vi "ConnectFieldTestServer.vi"(0 "FileName(.txt)":string="Test", 1 "working directory":path=path "C:/RageATE-Pickerel/Automated Tests/Tetra_RFSM/support_files/FieldTestServer", 5 "error in (no error)":errorcluster, 6 "UseCmdFile(T)":bool, 7 "Skip(T)":bool, 11 "CmdWindowHide(T)":bool, 13 "OpenNewFt(T)":bool=TRUE) -> (10 "PID":string="3196", 12 "cmd_path_out":path=path "C:/RageATE-Pickerel/Automated Tests/Tetra_RFSM/support_files/FieldTestServer/cmd /c FieldTest.exe testConfig_RfsmOnly.scn > Test.txt", 14 "success?(t)":bool=TRUE, 16 "connectToFt":string, 17 "cctFt error":string, 18 "cctFt output":string, 19 "error out":errorcluster)   [LabVIEW 2018]
panel:
  out "FtSvcOpen?(t)":bool
  out "KillFT(t)":bool caption="OK"
  out "FieldTestOpen?(t)":bool
  out "standard output":string="INFO: No tasks are running which match the specified criteria.Image Name                     PID Services                                    \r\n========================= ======== ============================================\r\nSystem Idle Process              0 N/A                                         \r\nSystem                           4 N/A                                         \r\nRegistry                       124 N/A                                         \r\nsmss.exe                       452 N/A                                         \r\ncsrss.exe                      592 N/A                                         \r\nwininit.exe                    792 N/A                                         \r\ncsrss.exe                      800 N/A                                         \r\nservices.exe                   880 N/A                                         \r\nlsass.exe                      888 KeyIso, SamSs, VaultSvc                     \r\nsvchost.exe                     84 BrokerInfrastructure, DcomLaunch, PlugPlay, \r\n                                   Power, SystemEventsBroker                   \r\nfontdrvhost.exe                536 N/A                                         \r\nwinlogon.exe                   664 N/A                                         \r\nfontdrvhost.exe                732 N/A                                         \r\nsvchost.exe                    964 RpcEptMapper, RpcSs                         \r\nsvchost.exe                    708 LSM                                         \r\ndwm.exe                       1080 N/A                                         \r\nsvchost.exe                   1276 NcbService                                  \r\nsvchost.exe                   1316 lmhosts                                     \r\nsvchost.exe                   1324 TimeBrokerSvc                               \r\nsvchost.exe                   1388 EventLog                                    \r\nsvchost.exe                   1396 hidserv                                     \r\nsvchost.exe                   1544 DevQueryBroker                              \r\nsvchost.exe                   1552 nsi                                         \r\nsvchost.exe                   1608 Dhcp                                        \r\nNVDisplay.Container.exe       1736 NVDisplay.ContainerLocalSystem              \r\nsvchost.exe                   1752 NlaSvc                                      \r\nsvchost.exe                   1812 Schedule                                    \r\nsvchost.exe                   1900 ProfSvc                                     \r\nsvchost.exe                   1908 SysMain                                     \r\nsvchost.exe                   1916 Themes                                      \r\nsvchost.exe                   1924 netprofm                                    \r\nsvchost.exe                   1940 EventSystem                                 \r\nsvchost.exe                   2052 SENS                                        \r\nsvchost.exe                   2076 AudioEndpointBuilder                        \r\nsvchost.exe                   2084 FontCache                                   \r\nMemory Compression            2144 N/A                                         \r\nsvchost.exe                   2456 WinHttpAutoProxySvc                         \r\nsvchost.exe                   2472 UserManager                                 \r\nsvchost.exe                   2532 Dnscache                                    \r\nsvchost.exe                   2612 Audiosrv                                    \r\nsvchost.exe                   2664 Wcmsvc                                      \r\nsvchost.exe                   2672 DusmSvc                                     \r\nsvchost.exe                   2736 ShellHWDetection                            \r\nspoolsv.exe                   2912 Spooler                                     \r\nsvchost.exe                   2956 BFE, mpssvc                                 \r\nsvchost.exe                   2996 StateRepository                             \r\nsvchost.exe                   3032 LanmanWorkstation                           \r\nsvchost.exe                   3260 CoreMessagingRegistrar                      \r\nsvchost.exe                   3268 CryptSvc                                    \r\nsvchost.exe                   3276 TermService                                 \r\nsvchost.exe                   3284 Winmgmt                                     \r\nsvchost.exe                   3292 DiagTrack                                   \r\nsvchost.exe                   3300 DPS                                         \r\nsvchost.exe                   3308 WpnService                                  \r\nIOLibrariesService.exe        3316 IOLibrariesService                          \r\nsvchost.exe                   3332 TrkWks                                      \r\nsvchost.exe                   3340 stisvc                                      \r\nnipalsm.exe                   3352 ni488enumsvc                                \r\nnimxs.exe                     3360 mxssvr                                      \r\nsvchost.exe                   3372 SstpSvc                                     \r\nKeysightCommunicationsFab     3380 KeysightCommunicationsFabric                \r\nLegacyDiscoveryService.ex     3392 AgilentInstrumentDiscoveryService           \r\nsvchost.exe                   3408 DeviceAssociationService                    \r\nLxiMdnsResponder.exe          3416 AgtMdnsResponder                            \r\nKeysightInstrumentIoServi     3460 KeysightInstrumentIoService                 \r\nnisvcloc.exe                  3484 NiSvcLoc                                    \r\ntvnserver.exe                 3496 tvnserver                                   \r\nnipxicms.exe                  3508 nipxicmsvc                                  \r\nnisds.exe                     3536 nisds                                       \r\narmsvc.exe                    3548 AdobeARMservice                             \r\nMsMpEng.exe                   3556 WinDefend                                   \r\nvss-service-x64.exe           3568 Synology Drive VSS Service x64              \r\nniauth_daemon.exe             3588 niauth                                      \r\nOfficeClickToRun.exe          3772 ClickToRunSvc                               \r\nsvchost.exe                   3808 WdiServiceHost                              \r\ndasHost.exe                   3940 N/A                                         \r\nsvchost.exe                   3984 iphlpsvc                                    \r\nHppSupportService.exe         4036 HppSupportService                           \r\nAgilentLicenseService.exe     4044 Agilent License Service                     \r\nsvchost.exe                   4076 LanmanServer                                \r\nsvchost.exe                   3976 RasMan                                      \r\nkiis-service.exe              4372 N/A                                         \r\nconhost.exe                   4388 N/A                                         \r\nsvchost.exe                   4748 SSDPSRV                                     \r\nlkads.exe                     4800 lkClassAds                                  \r\nniroco.exe                    4808 niroco                                      \r\nlktsrv.exe                    4964 lkTimeSync                                  \r\nnipxism.exe                   4972 nipxirmu                                    \r\nnidmsrv.exe                   4992 NIDomainService                             \r\nnimdnsResponder.exe           5008 nimDNSResponder                             \r\nnidevldu.exe                  5124 nidevldu                                    \r\ntagsrv.exe                    5184 NITaggerService                             \r\nniLxiDiscovery.exe            5252 niLXIDiscovery                              \r\nniDiscSvc.exe                 5276 NINetworkDiscovery                          \r\nsvchost.exe                   5452 PolicyAgent                                 \r\ndasHost.exe                   6020 N/A                                         \r\nLegacyIOLibrariesService.     6084 AgilentIOLibrariesService                   \r\nConnectionExpert.Server.H     6092 KeysightInstrumentDiscoveryService          \r\nSystemWebServer.exe           6108 NISystemWebServer                           \r\nApplicationWebServer.exe      6564 NIApplicationWebServer                      \r\nNIWebServiceContainer.exe     6572 N/A                                         \r\nNIWebServiceContainer.exe     6648 N/A                                         \r\nNIWebServiceContainer.exe     6708 N/A                                         \r\nNIWebServiceContainer.exe     6776 N/A                                         \r\nsvchost.exe                   7132 DispBrokerDesktopSvc                        \r\nsvchost.exe                   6716 NcdAutoSetup                                \r\nsvchost.exe                   6916 FDResPub                                    \r\nNIWebServiceContainer.exe     6060 N/A                                         \r\nIolsNkoServer.exe             2908 N/A                                         \r\nSearchIndexer.exe             6980 WSearch                                     \r\niproc488.exe                  7688 N/A                                         \r\niproc82357.exe                7764 N/A                                         \r\niproc389.exe                  7800 N/A                                         \r\nsecure-config-service.exe     7844 N/A                                         \r\nconhost.exe                   7852 N/A                                         \r\nAggregatorHost.exe            7504 N/A                                         \r\nIolsPXIResourceManager.ex     8104 IolsPXIResourceManager                      \r\nsecurity-comm-hpp-microse     7252 N/A                                         \r\nconhost.exe                   7296 N/A                                         \r\ndllhost.exe                   8820 N/A                                         \r\nNisSrv.exe                    9092 WdNisSvc                                    \r\nsvchost.exe                   8212 WdiSystemHost                               \r\nsvchost.exe                   7508 PcaSvc                                      \r\nNVDisplay.Container.exe       9456 N/A                                         \r\nsvchost.exe                   2932 DoSvc                                       \r\nsvchost.exe                   7572 RmSvc                                       \r\nsvchost.exe                   1420 StorSvc                                     \r\nsvchost.exe                   9584 NgcSvc                                      \r\nsvchost.exe                   9784 NgcCtnrSvc                                  \r\nsvchost.exe                   9676 CertPropSvc                                 \r\nsvchost.exe                   9640 SCardSvr                                    \r\nsvchost.exe                   2564 CDPSvc                                      \r\nSgrmBroker.exe                1568 SgrmBroker                                  \r\nuhssvc.exe                    2040 uhssvc                                      \r\nsvchost.exe                   2604 TokenBroker                                 \r\nsvchost.exe                   2936 UsoSvc                                      \r\nsvchost.exe                   3600 W32Time                                     \r\nsvchost.exe                   4356 wscsvc                                      \r\nsvchost.exe                   1288 InstallService                              \r\nsihost.exe                    8492 N/A                                         \r\nsvchost.exe                   9356 CDPUserSvc_5dc012                           \r\nsvchost.exe                    896 WpnUserService_5dc012                       \r\ntaskhostw.exe                 4328 N/A                                         \r\nsvchost.exe                   2420 TabletInputService                          \r\nctfmon.exe                    2864 N/A                                         \r\nexplorer.exe                  2108 N/A                                         \r\nsvchost.exe                   7040 camsvc                                      \r\nsvchost.exe                   9196 cbdhsvc_5dc012                              \r\nStartMenuExperienceHost.e      704 N/A                                         \r\nRuntimeBroker.exe             2356 N/A                                         \r\nSearchApp.exe                10092 N/A                                         \r\nRuntimeBroker.exe             8364 N/A                                         \r\nsvchost.exe                   8024 LicenseManager                              \r\nRuntimeBroker.exe            11248 N/A                                         \r\nsvchost.exe                  10560 OneSyncSvc_5dc012,                          \r\n                                   PimIndexMaintenanceSvc_5dc012,              \r\n                                   UnistoreSvc_5dc012, UserDataSvc_5dc012      \r\nPhoneExperienceHost.exe       9244 N/A                                         \r\ndllhost.exe                  11364 N/A                                         \r\nRuntimeBroker.exe            11520 N/A                                         \r\nTextInputHost.exe            11604 N/A                                         \r\nSecurityHealthSystray.exe    11752 N/A                                         \r\nSecurityHealthService.exe    11784 SecurityHealthService                       \r\ntvnserver.exe                11908 N/A                                         \r\nsvchost.exe                  12676 Appinfo                                     \r\nms-teams.exe                  9444 N/A                                         \r\nRuntimeBroker.exe             6580 N/A                                         \r\niprocsvr.exe                  7308 N/A                                         \r\niproc8491.exe                 6028 N/A                                         \r\nAgilentLicenseNotifier.ex    12968 N/A                                         \r\nDeviceMonitor.exe            13488 N/A                                         \r\nmsedgewebview2.exe           13624 N/A                                         \r\ndllhost.exe                  13660 N/A                                         \r\nmsedgewebview2.exe           13680 N/A                                         \r\nmsedgewebview2.exe           13996 N/A                                         \r\nmsedgewebview2.exe           14016 N/A                                         \r\nmsedgewebview2.exe           14040 N/A                                         \r\nmsedgewebview2.exe           14156 N/A                                         \r\nnierserver.exe               13372 N/A                                         \r\ncloud-drive-ui.exe           15264 N/A                                         \r\ncloud-drive-connect.exe       8788 N/A                                         \r\nconhost.exe                  14372 N/A                                         \r\ncloud-drive-daemon.exe       15008 N/A                                         \r\nconhost.exe                  15052 N/A                                         \r\nmsedgewebview2.exe           14456 N/A                                         \r\nsvchost.exe                  14524 lfsvc                                       \r\nApplicationFrameHost.exe     12392 N/A                                         \r\nCalculatorApp.exe            12440 N/A                                         \r\nRuntimeBroker.exe             3492 N/A                                         \r\nSystemSettings.exe            3580 N/A                                         \r\nUserOOBEBroker.exe           12412 N/A                                         \r\nMicrosoft.Media.Player.ex     6192 N/A                                         \r\nRuntimeBroker.exe             1724 N/A                                         \r\nOUTLOOK.EXE                   3908 N/A                                         \r\nai.exe                       10320 N/A                                         \r\nmsedgewebview2.exe            9184 N/A                                         \r\nmsedgewebview2.exe            2492 N/A                                         \r\nmsedgewebview2.exe            3016 N/A                                         \r\nmsedgewebview2.exe            1368 N/A                                         \r\nmsedgewebview2.exe           10564 N/A                                         \r\nmsedgewebview2.exe            7120 N/A                                         \r\nmsedgewebview2.exe           12888 N/A                                         \r\nfirefox.exe                  13096 N/A                                         \r\nfirefox.exe                  12984 N/A                                         \r\nfirefox.exe                  13228 N/A                                         \r\nfirefox.exe                   7624 N/A                                         \r\nfirefox.exe                   6244 N/A                                         \r\nfirefox.exe                  15312 N/A                                         \r\nfirefox.exe                    820 N/A                                         \r\nTGitCache.exe                 5360 N/A                                         \r\nsvchost.exe                  14784 wcncsvc                                     \r\nShellExperienceHost.exe      12404 N/A                                         \r\nRuntimeBroker.exe             6468 N/A                                         \r\nVideo.UI.exe                 13360 N/A                                         \r\nRuntimeBroker.exe            13412 N/A                                         \r\nsvchost.exe                   5304 BthAvctpSvc                                 \r\nsvchost.exe                   1264 WebClient                                   \r\nWinRAR.exe                   15756 N/A                                         \r\nmsedge.exe                    9240 N/A                                         \r\nmsedge.exe                   16444 N/A                                         \r\nmsedge.exe                   15112 N/A                                         \r\nmsedge.exe                   15656 N/A                                         \r\nmsedge.exe                    9208 N/A                                         \r\nmsedge.exe                    9068 N/A                                         \r\nmsedge.exe                   16896 N/A                                         \r\nmsedge.exe                   10192 N/A                                         \r\nmsedge.exe                   10844 N/A                                         \r\nmsedge.exe                    1432 N/A                                         \r\nmsedge.exe                   12940 N/A                                         \r\nmsedge.exe                    1652 N/A                                         \r\nmsedge.exe                    9800 N/A                                         \r\nmsedge.exe                   13316 N/A                                         \r\nmsedge.exe                   15800 N/A                                         \r\nmsedge.exe                   11328 N/A                                         \r\nmsedge.exe                    1808 N/A                                         \r\nfirefox.exe                  17812 N/A                                         \r\nfirefox.exe                  17620 N/A                                         \r\nfirefox.exe                  14588 N/A                                         \r\nmsedge.exe                   11468 N/A                                         \r\nai.exe                       15952 N/A                                         \r\nmsedge.exe                    5872 N/A                                         \r\nmsedge.exe                   10824 N/A                                         \r\nSnippingTool.exe              4636 N/A                                         \r\ntvnviewer.exe                18856 N/A                                         \r\nfirefox.exe                  14060 N/A                                         \r\nfirefox.exe                   2116 N/A                                         \r\nfirefox.exe                  10568 N/A                                         \r\nfirefox.exe                  15436 N/A                                         \r\nfirefox.exe                  10688 N/A                                         \r\nfirefox.exe                  15292 N/A                                         \r\nfirefox.exe                  19384 N/A                                         \r\nfirefox.exe                   1412 N/A                                         \r\nsvchost.exe                  15940 DsSvc                                       \r\nfirefox.exe                   3848 N/A                                         \r\nfirefox.exe                  12172 N/A                                         \r\nfirefox.exe                  10924 N/A                                         \r\naudiodg.exe                   9120 N/A                                         \r\nOneDrive.exe                  9532 N/A                                         \r\nMicrosoft.SharePoint.exe     15608 N/A                                         \r\nFileCoAuth.exe               13268 N/A                                         \r\nLabVIEW.exe                  17668 N/A                                         \r\nnimxsoffline.exe             10864 N/A                                         \r\nfirefox.exe                  18416 N/A                                         \r\nfirefox.exe                  12188 N/A                                         \r\nWmiPrvSE.exe                 17864 N/A                                         \r\nsvchost.exe                  17244 gpsvc                                       \r\nsmartscreen.exe              17352 N/A                                         \r\nSearchProtocolHost.exe        3472 N/A                                         \r\nSearchFilterHost.exe         12868 N/A                                         \r\ntasklist.exe                 19020 N/A                                         \r\nconhost.exe                  18652 N/AImage Name                     PID Services                                    \r\n========================= ======== ============================================\r\nSystem Idle Process              0 N/A                                         \r\nSystem                           4 N/A                                         \r\nRegistry                       124 N/A                                         \r\nsmss.exe                       452 N/A                                         \r\ncsrss.exe                      592 N/A                                         \r\nwininit.exe                    792 N/A                                         \r\ncsrss.exe                      800 N/A                                         \r\nservices.exe                   880 N/A                                         \r\nlsass.exe                      888 KeyIso, SamSs, VaultSvc                     \r\nsvchost.exe                     84 BrokerInfrastructure, DcomLaunch, PlugPlay, \r\n                                   Power, SystemEventsBroker                   \r\nfontdrvhost.exe                536 N/A                                         \r\nwinlogon.exe                   664 N/A                                         \r\nfontdrvhost.exe                732 N/A                                         \r\nsvchost.exe                    964 RpcEptMapper, RpcSs                         \r\nsvchost.exe                    708 LSM                                         \r\ndwm.exe                       1080 N/A                                         \r\nsvchost.exe                   1276 NcbService                                  \r\nsvchost.exe                   1316 lmhosts                                     \r\nsvchost.exe                   1324 TimeBrokerSvc                               \r\nsvchost.exe                   1388 EventLog                                    \r\nsvchost.exe                   1396 hidserv                                     \r\nsvchost.exe                   1544 DevQueryBroker                              \r\nsvchost.exe                   1552 nsi                                         \r\nsvchost.exe                   1608 Dhcp                                        \r\nNVDisplay.Container.exe       1736 NVDisplay.ContainerLocalSystem              \r\nsvchost.exe                   1752 NlaSvc                                      \r\nsvchost.exe                   1812 Schedule                                    \r\nsvchost.exe                   1900 ProfSvc                                     \r\nsvchost.exe                   1908 SysMain                                     \r\nsvchost.exe                   1916 Themes                                      \r\nsvchost.exe                   1924 netprofm                                    \r\nsvchost.exe                   1940 EventSystem                                 \r\nsvchost.exe                   2052 SENS                                        \r\nsvchost.exe                   2076 AudioEndpointBuilder                        \r\nsvchost.exe                   2084 FontCache                                   \r\nMemory Compression            2144 N/A                                         \r\nsvchost.exe                   2456 WinHttpAutoProxySvc                         \r\nsvchost.exe                   2472 UserManager                                 \r\nsvchost.exe                   2532 Dnscache                                    \r\nsvchost.exe                   2612 Audiosrv                                    \r\nsvchost.exe                   2664 Wcmsvc                                      \r\nsvchost.exe                   2672 DusmSvc                                     \r\nsvchost.exe                   2736 ShellHWDetection                            \r\nspoolsv.exe                   2912 Spooler                                     \r\nsvchost.exe                   2956 BFE, mpssvc                                 \r\nsvchost.exe                   2996 StateRepository                             \r\nsvchost.exe                   3032 LanmanWorkstation                           \r\nsvchost.exe                   3260 CoreMessagingRegistrar                      \r\nsvchost.exe                   3268 CryptSvc                                    \r\nsvchost.exe                   3276 TermService                                 \r\nsvchost.exe                   3284 Winmgmt                                     \r\nsvchost.exe                   3292 DiagTrack                                   \r\nsvchost.exe                   3300 DPS                                         \r\nsvchost.exe                   3308 WpnService                                  \r\nIOLibrariesService.exe        3316 IOLibrariesService                          \r\nsvchost.exe                   3332 TrkWks                                      \r\nsvchost.exe                   3340 stisvc                                      \r\nnipalsm.exe                   3352 ni488enumsvc                                \r\nnimxs.exe                     3360 mxssvr                                      \r\nsvchost.exe                   3372 SstpSvc                                     \r\nKeysightCommunicationsFab     3380 KeysightCommunicationsFabric                \r\nLegacyDiscoveryService.ex     3392 AgilentInstrumentDiscoveryService           \r\nsvchost.exe                   3408 DeviceAssociationService                    \r\nLxiMdnsResponder.exe          3416 AgtMdnsResponder                            \r\nKeysightInstrumentIoServi     3460 KeysightInstrumentIoService                 \r\nnisvcloc.exe                  3484 NiSvcLoc                                    \r\ntvnserver.exe                 3496 tvnserver                                   \r\nnipxicms.exe                  3508 nipxicmsvc                                  \r\nnisds.exe                     3536 nisds                                       \r\narmsvc.exe                    3548 AdobeARMservice                             \r\nMsMpEng.exe                   3556 WinDefend                                   \r\nvss-service-x64.exe           3568 Synology Drive VSS Service x64              \r\nniauth_daemon.exe             3588 niauth                                      \r\nOfficeClickToRun.exe          3772 ClickToRunSvc                               \r\nsvchost.exe                   3808 WdiServiceHost                              \r\ndasHost.exe                   3940 N/A                                         \r\nsvchost.exe                   3984 iphlpsvc                                    \r\nHppSupportService.exe         4036 HppSupportService                           \r\nAgilentLicenseService.exe     4044 Agilent License Service                     \r\nsvchost.exe                   4076 LanmanServer                                \r\nsvchost.exe                   3976 RasMan                                      \r\nkiis-service.exe              4372 N/A                                         \r\nconhost.exe                   4388 N/A                                         \r\nsvchost.exe                   4748 SSDPSRV                                     \r\nlkads.exe                     4800 lkClassAds                                  \r\nniroco.exe                    4808 niroco                                      \r\nlktsrv.exe                    4964 lkTimeSync                                  \r\nnipxism.exe                   4972 nipxirmu                                    \r\nnidmsrv.exe                   4992 NIDomainService                             \r\nnimdnsResponder.exe           5008 nimDNSResponder                             \r\nnidevldu.exe                  5124 nidevldu                                    \r\ntagsrv.exe                    5184 NITaggerService                             \r\nniLxiDiscovery.exe            5252 niLXIDiscovery                              \r\nniDiscSvc.exe                 5276 NINetworkDiscovery                          \r\nsvchost.exe                   5452 PolicyAgent                                 \r\ndasHost.exe                   6020 N/A                                         \r\nLegacyIOLibrariesService.     6084 AgilentIOLibrariesService                   \r\nConnectionExpert.Server.H     6092 KeysightInstrumentDiscoveryService          \r\nSystemWebServer.exe           6108 NISystemWebServer                           \r\nApplicationWebServer.exe      6564 NIApplicationWebServer                      \r\nNIWebServiceContainer.exe     6572 N/A                                         \r\nNIWebServiceContainer.exe     6648 N/A                                         \r\nNIWebServiceContainer.exe     6708 N/A                                         \r\nNIWebServiceContainer.exe     6776 N/A                                         \r\nsvchost.exe                   7132 DispBrokerDesktopSvc                        \r\nsvchost.exe                   6716 NcdAutoSetup                                \r\nsvchost.exe                   6916 FDResPub                                    \r\nNIWebServiceContainer.exe     6060 N/A                                         \r\nIolsNkoServer.exe             2908 N/A                                         \r\nSearchIndexer.exe             6980 WSearch                                     \r\niproc488.exe                  7688 N/A                                         \r\niproc82357.exe                7764 N/A                                         \r\niproc389.exe                  7800 N/A                                         \r\nsecure-config-service.exe     7844 N/A                                         \r\nconhost.exe                   7852 N/A                                         \r\nAggregatorHost.exe            7504 N/A                                         \r\nIolsPXIResourceManager.ex     8104 IolsPXIResourceManager                      \r\nsecurity-comm-hpp-microse     7252 N/A                                         \r\nconhost.exe                   7296 N/A                                         \r\ndllhost.exe                   8820 N/A                                         \r\nNisSrv.exe                    9092 WdNisSvc                                    \r\nsvchost.exe                   8212 WdiSystemHost                               \r\nsvchost.exe                   7508 PcaSvc                                      \r\nNVDisplay.Container.exe       9456 N/A                                         \r\nsvchost.exe                   2932 DoSvc                                       \r\nsvchost.exe                   7572 RmSvc                                       \r\nsvchost.exe                   1420 StorSvc                                     \r\nsvchost.exe                   9584 NgcSvc                                      \r\nsvchost.exe                   9784 NgcCtnrSvc                                  \r\nsvchost.exe                   9676 CertPropSvc                                 \r\nsvchost.exe                   9640 SCardSvr                                    \r\nsvchost.exe                   2564 CDPSvc                                      \r\nSgrmBroker.exe                1568 SgrmBroker                                  \r\nuhssvc.exe                    2040 uhssvc                                      \r\nsvchost.exe                   2604 TokenBroker                                 \r\nsvchost.exe                   2936 UsoSvc                                      \r\nsvchost.exe                   3600 W32Time                                     \r\nsvchost.exe                   4356 wscsvc                                      \r\nsvchost.exe                   1288 InstallService                              \r\nsihost.exe                    8492 N/A                                         \r\nsvchost.exe                   9356 CDPUserSvc_5dc012                           \r\nsvchost.exe                    896 WpnUserService_5dc012                       \r\ntaskhostw.exe                 4328 N/A                                         \r\nsvchost.exe                   2420 TabletInputService                          \r\nctfmon.exe                    2864 N/A                                         \r\nexplorer.exe                  2108 N/A                                         \r\nsvchost.exe                   7040 camsvc                                      \r\nsvchost.exe                   9196 cbdhsvc_5dc012                              \r\nStartMenuExperienceHost.e      704 N/A                                         \r\nRuntimeBroker.exe             2356 N/A                                         \r\nSearchApp.exe                10092 N/A                                         \r\nRuntimeBroker.exe             8364 N/A                                         \r\nsvchost.exe                   8024 LicenseManager                              \r\nRuntimeBroker.exe            11248 N/A                                         \r\nsvchost.exe                  10560 OneSyncSvc_5dc012,                          \r\n                                   PimIndexMaintenanceSvc_5dc012,              \r\n                                   UnistoreSvc_5dc012, UserDataSvc_5dc012      \r\nPhoneExperienceHost.exe       9244 N/A                                         \r\ndllhost.exe                  11364 N/A                                         \r\nRuntimeBroker.exe            11520 N/A                                         \r\nTextInputHost.exe            11604 N/A                                         \r\nSecurityHealthSystray.exe    11752 N/A                                         \r\nSecurityHealthService.exe    11784 SecurityHealthService                       \r\ntvnserver.exe                11908 N/A                                         \r\nsvchost.exe                  12676 Appinfo                                     \r\nms-teams.exe                  9444 N/A                                         \r\nRuntimeBroker.exe             6580 N/A                                         \r\niprocsvr.exe                  7308 N/A                                         \r\niproc8491.exe                 6028 N/A                                         \r\nAgilentLicenseNotifier.ex    12968 N/A                                         \r\nDeviceMonitor.exe            13488 N/A                                         \r\nmsedgewebview2.exe           13624 N/A                                         \r\ndllhost.exe                  13660 N/A                                         \r\nmsedgewebview2.exe           13680 N/A                                         \r\nmsedgewebview2.exe           13996 N/A                                         \r\nmsedgewebview2.exe           14016 N/A                                         \r\nmsedgewebview2.exe           14040 N/A                                         \r\nmsedgewebview2.exe           14156 N/A                                         \r\nnierserver.exe               13372 N/A                                         \r\ncloud-drive-ui.exe           15264 N/A                                         \r\ncloud-drive-connect.exe       8788 N/A                                         \r\nconhost.exe                  14372 N/A                                         \r\ncloud-drive-daemon.exe       15008 N/A                                         \r\nconhost.exe                  15052 N/A                                         \r\nmsedgewebview2.exe           14456 N/A                                         \r\nsvchost.exe                  14524 lfsvc                                       \r\nApplicationFrameHost.exe     12392 N/A                                         \r\nCalculatorApp.exe            12440 N/A                                         \r\nRuntimeBroker.exe             3492 N/A                                         \r\nSystemSettings.exe            3580 N/A                                         \r\nUserOOBEBroker.exe           12412 N/A                                         \r\nMicrosoft.Media.Player.ex     6192 N/A                                         \r\nRuntimeBroker.exe             1724 N/A                                         \r\nOUTLOOK.EXE                   3908 N/A                                         \r\nai.exe                       10320 N/A                                         \r\nmsedgewebview2.exe            9184 N/A                                         \r\nmsedgewebview2.exe            2492 N/A                                         \r\nmsedgewebview2.exe            3016 N/A                                         \r\nmsedgewebview2.exe            1368 N/A                                         \r\nmsedgewebview2.exe           10564 N/A                                         \r\nmsedgewebview2.exe            7120 N/A                                         \r\nmsedgewebview2.exe           12888 N/A                                         \r\nfirefox.exe                  13096 N/A                                         \r\nfirefox.exe                  12984 N/A                                         \r\nfirefox.exe                  13228 N/A                                         \r\nfirefox.exe                   7624 N/A                                         \r\nfirefox.exe                   6244 N/A                                         \r\nfirefox.exe                  15312 N/A                                         \r\nfirefox.exe                    820 N/A                                         \r\nTGitCache.exe                 5360 N/A                                         \r\nsvchost.exe                  14784 wcncsvc                                     \r\nShellExperienceHost.exe      12404 N/A                                         \r\nRuntimeBroker.exe             6468 N/A                                         \r\nVideo.UI.exe                 13360 N/A                                         \r\nRuntimeBroker.exe            13412 N/A                                         \r\nsvchost.exe                   5304 BthAvctpSvc                                 \r\nsvchost.exe                   1264 WebClient                                   \r\nWinRAR.exe                   15756 N/A                                         \r\nmsedge.exe                    9240 N/A                                         \r\nmsedge.exe                   16444 N/A                                         \r\nmsedge.exe                   15112 N/A                                         \r\nmsedge.exe                   15656 N/A                                         \r\nmsedge.exe                    9208 N/A                                         \r\nmsedge.exe                    9068 N/A                                         \r\nmsedge.exe                   16896 N/A                                         \r\nmsedge.exe                   10192 N/A                                         \r\nmsedge.exe                   10844 N/A                                         \r\nmsedge.exe                    1432 N/A                                         \r\nmsedge.exe                   12940 N/A                                         \r\nmsedge.exe                    1652 N/A                                         \r\nmsedge.exe                    9800 N/A                                         \r\nmsedge.exe                   13316 N/A                                         \r\nmsedge.exe                   15800 N/A                                         \r\nmsedge.exe                   11328 N/A                                         \r\nmsedge.exe                    1808 N/A                                         \r\nfirefox.exe                  17812 N/A                                         \r\nfirefox.exe                  17620 N/A                                         \r\nfirefox.exe                  14588 N/A                                         \r\nmsedge.exe                   11468 N/A                                         \r\nai.exe                       15952 N/A                                         \r\nmsedge.exe                    5872 N/A                                         \r\nmsedge.exe                   10824 N/A                                         \r\nSnippingTool.exe              4636 N/A                                         \r\ntvnviewer.exe                18856 N/A                                         \r\nfirefox.exe                  14060 N/A                                         \r\nfirefox.exe                   2116 N/A                                         \r\nfirefox.exe                  10568 N/A                                         \r\nfirefox.exe                  15436 N/A                                         \r\nfirefox.exe                  10688 N/A                                         \r\nfirefox.exe                  15292 N/A                                         \r\nfirefox.exe                  19384 N/A                                         \r\nfirefox.exe                   1412 N/A                                         \r\nsvchost.exe                  15940 DsSvc                                       \r\nfirefox.exe                   3848 N/A                                         \r\nfirefox.exe                  12172 N/A                                         \r\nfirefox.exe                  10924 N/A                                         \r\naudiodg.exe                   9120 N/A                                         \r\nOneDrive.exe                  9532 N/A                                         \r\nMicrosoft.SharePoint.exe     15608 N/A                                         \r\nFileCoAuth.exe               13268 N/A                                         \r\nLabVIEW.exe                  17668 N/A                                         \r\nnimxsoffline.exe             10864 N/A                                         \r\nfirefox.exe                  18416 N/A                                         \r\nfirefox.exe                  12188 N/A                                         \r\nWmiPrvSE.exe                 17864 N/A                                         \r\nsvchost.exe                  17244 gpsvc                                       \r\nsmartscreen.exe              17352 N/A                                         \r\nSearchProtocolHost.exe        3472 N/A                                         \r\nSearchFilterHost.exe         12868 N/A                                         \r\ncmd.exe                      17900 N/A                                         \r\ntasklist.exe                 16772 N/A                                         \r\nconhost.exe                  18564 N/A                                         \r\nconhost.exe                   4840 N/A                                         \r\nFieldTest.exe                 3196 N/A"
  # "This vi will kill running instance of FieldTest, and open a fresh instance.\nFileName = File created that cmd line is written to, IF \"UseCmdFile\" is checked\nCmdWindowHide = T, will run the window not visible so it cant be messed with."
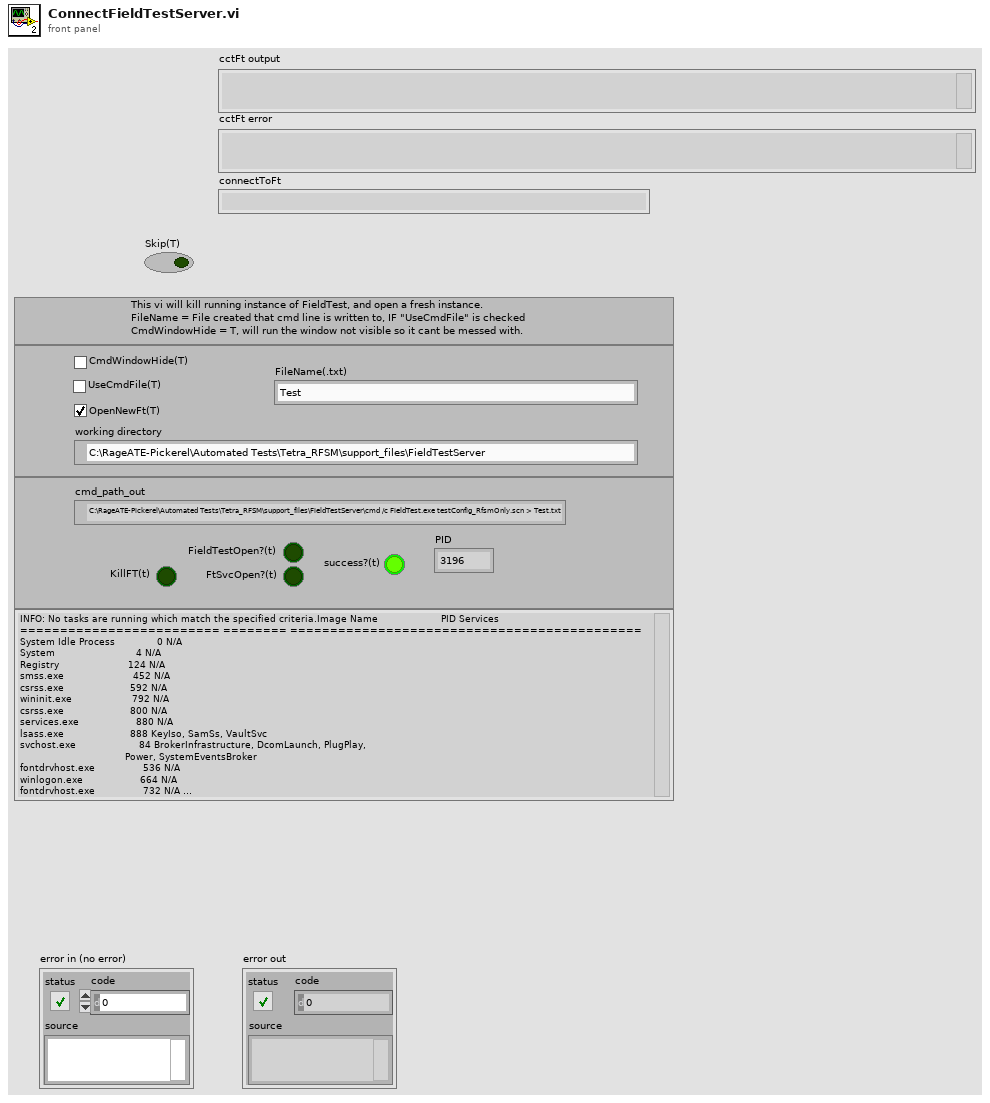
[diagram p1: front panel]
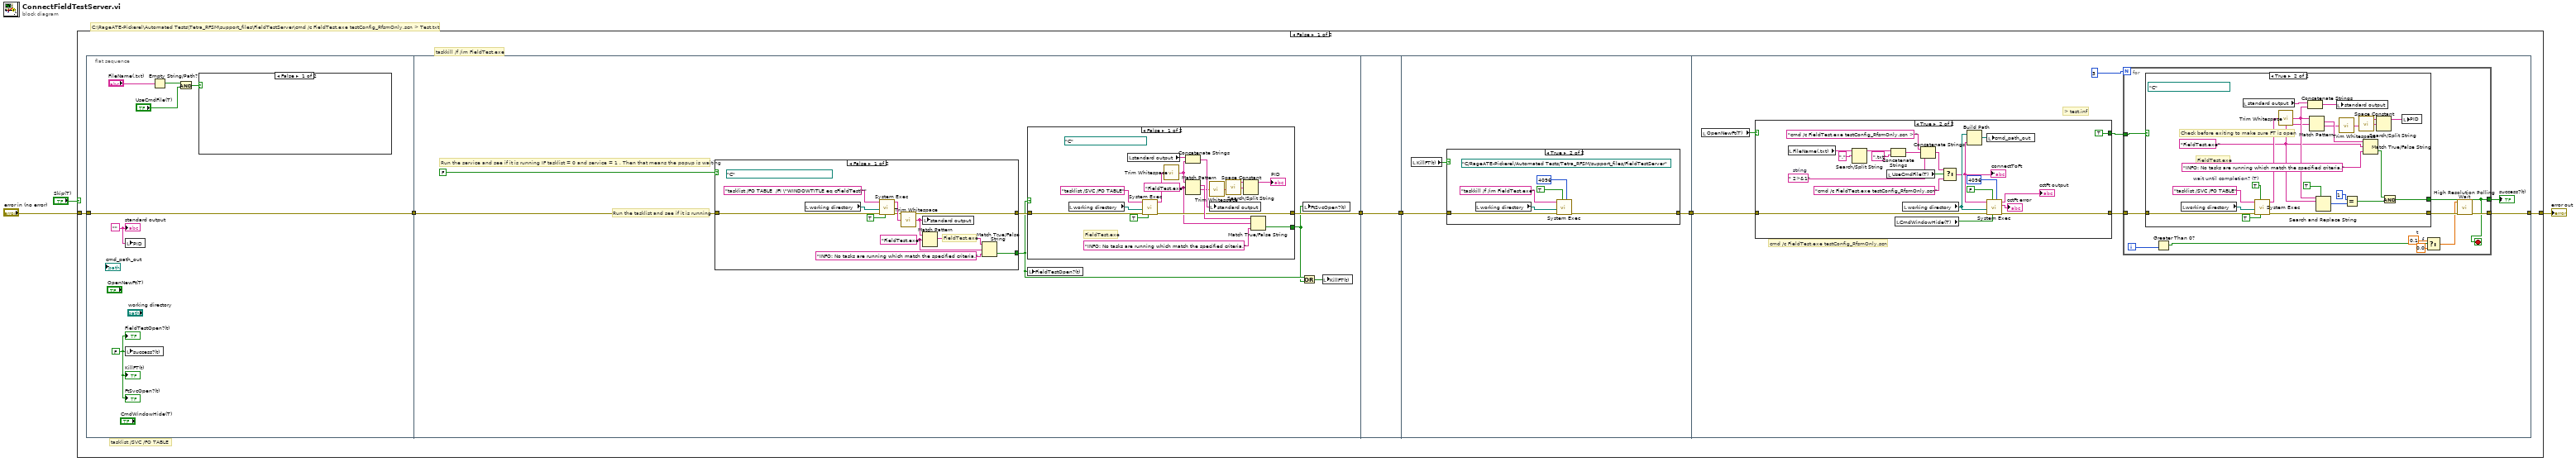
[diagram p0: block diagram]
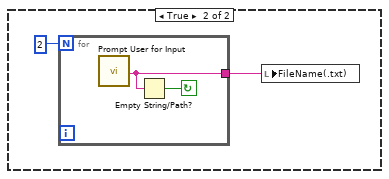
[diagram p2: hidden frame]
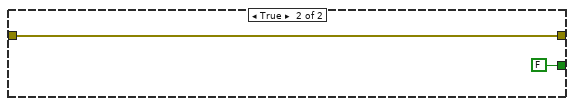
[diagram p3: hidden frame]
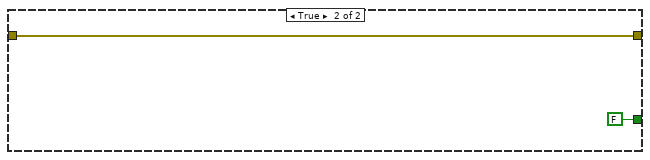
[diagram p4: hidden frame]
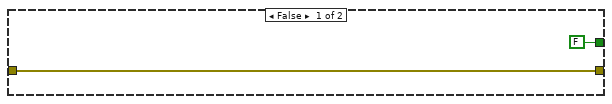
[diagram p6: hidden frame]
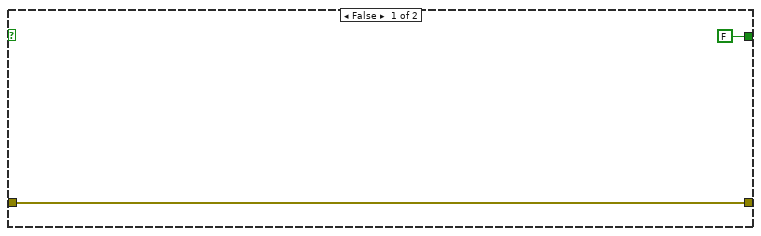
[diagram p7: hidden frame]
diagram:
  # "C:\\RageATE-Pickerel\\Automated Tests\\Tetra_RFSM\\support_files\\FieldTestServer\\cmd /c FieldTest.exe testConfig_RfsmOnly.scn > Test.txt"
  n1 = case shown="False" "Skip(T)" {
    tunnel: [w5 w136] -> w3
    tunnel: "error in (no error)" -> [w4 w136]
    frame False {
      # "tasklist /SVC /FO TABLE"
      # "taskkill /f /im FieldTest.exe"
      n2 = flat-sequence {
        tunnel: [w16] -> w9
        tunnel: w4 -> [w16]
        tunnel: w9 -> [w27]
        tunnel: [w25] -> w8
        tunnel: [w60] -> w7
        tunnel: w8 -> [w60]
        tunnel: [w62] -> w6
        tunnel: w7 -> [w63]
        tunnel: [w77] -> w5
        tunnel: w6 -> [w76]
        frame #0 {
          w10 = FALSE ("OpenNewFT(t)")
          w15 = ""
          n3 = local write "PID"(w15) -> ()
          n4 = local write "success?(t)"(w10) -> ()
          n5 = Empty String/Path?(string/path="FileName(.txt)") -> (empty?=w14:bool)
          n6 = And(x=w14, y="UseCmdFile(T)") -> (x .and. y?=w13:bool)
          n7 = case shown="False" w13 {
            frame False {
            }
            frame True {
              n8 = for {
                N: 2 -> [_]
                tunnel: [w19] -> w17
                stop <- w20 continue-if-true
                n9 = call "Prompt User for Input"() -> ("File"=w19:string)  [unwired: 17 in, 2 out]
                n10 = Empty String/Path?(string/path=w19) -> (empty?=w20:bool)
              }
              n11 = local write "FileName(.txt)"(w17) -> ()
            }
          }
          "standard output" <- w15
          "FieldTestOpen?(t)" <- w10
          "KillFT(t)" <- w10
          "FtSvcOpen?(t)" <- w10
        }
        frame #1 {
          # "Run the service and see if it is running IF tasklist = 0 and service = 1 , Then that means the popup is waiting"
          # "Run the tasklist and see if it is running"
          n12 = case shown="False" FALSE {
            tunnel: [w54 FALSE ("selection")] -> w23
            tunnel: w27 -> [w50 w59]
            tunnel: [w49 w59] -> w26
            frame False {
              w52 = "FieldTest.exe" ("string")
              (unwired) path "C:/" ("working directory")
              # "FieldTest.exe"
              n13 = local read "working directory"() -> (w47:path)
              n14 = call <vilib>:"System Exec.vi"("run minimized? (F)"=TRUE, "error in (no error)"=w50, "working directory"=w47, "command line"="tasklist /FO TABLE  /FI \"WINDOWTITLE eq cFieldTest\"") -> ("error out"=w49:errorcluster, "standard output"=w57:string)  [unwired: 4 in, 2 out]
              n15 = call <vilib>:"Trim Whitespace.vi"("string"=w57) -> ("trimmed string"=w48:string)  [unwired: 1 in]
              n16 = local write "standard output"(w48) -> ()
              n17 = Match Pattern(string=w48, regular expression=w52) -> (match substring=w51:string)  [unwired: 1 in, 3 out]
              n18 = Match True/False String(2:"INFO: No tasks are running which match the specified criteria." ("false string"), 3:w52, 4:w51) -> (0:w54:bool)  [unwired: 1 out]
            }
            frame True {
            }
          }
          n19 = case shown="False" w23 {
            tunnel: [w41 FALSE ("selection")] -> w22
            tunnel: w26 -> [w38 w46]
            tunnel: [w37 w46] -> w25
            frame False {
              w33 = "FieldTest.exe" ("string")
              (unwired) path "C:/" ("working directory")
              # "FieldTest.exe"
              n20 = local read "working directory"() -> (w28:path)
              n21 = local read "standard output"() -> (w35:string)
              n22 = call <vilib>:"System Exec.vi"("run minimized? (F)"=TRUE, "error in (no error)"=w38, "working directory"=w28, "command line"="tasklist /SVC /FO TABLE") -> ("error out"=w37:errorcluster, "standard output"=w44:string)  [unwired: 4 in, 2 out]
              n23 = call <vilib>:"Trim Whitespace.vi"("string"=w44) -> ("trimmed string"=w34:string)  [unwired: 1 in]
              n24 = Concatenate Strings(w35, w34) -> (w36:string)
              n25 = Match Pattern(string=w34, regular expression=w33) -> (match substring=w39:string, after substring=w32:string)  [unwired: 1 in, 2 out]
              n26 = call <vilib>:"Trim Whitespace.vi"("string"=w32) -> ("trimmed string"=w31:string)  [unwired: 1 in]
              n27 = local write "standard output"(w36) -> ()
              n28 = call <vilib>:"Space Constant.vi"() -> ("String"=w30:string)
              n29 = Search/Split String(string=w31, search string/char (-)=w30) -> (substring before match=→"PID":string)  [unwired: 1 in, 2 out]
              n30 = Match True/False String(2:"INFO: No tasks are running which match the specified criteria." ("false string"), 3:w33, 4:w39) -> (0:w41:bool)  [unwired: 1 out]
            }
            frame True {
            }
          }
          n31 = local write "FieldTestOpen?(t)"(w23) -> ()
          n32 = Or(x=w23, y=w22) -> (x .or. y?=w21:bool)
          n33 = local write "FtSvcOpen?(t)"(w22) -> ()
          n34 = local write "KillFT(t)"(w21) -> ()
        }
        frame #2 {
        }
        frame #3 {
          n35 = local read "KillFT(t)"() -> (w61:bool)
          n36 = case shown="True" w61 {
            tunnel: w63 -> [w64 w69]
            tunnel: [w64 w68] -> w62
            frame False {
            }
            frame True {
              (unwired) path "C:/RageATE-Pickerel/Automated Tests/Tetra_RFSM/support_files/FieldTestServer" ("working directory")
              n37 = local read "working directory"() -> (w65:path)
              n38 = call <vilib>:"System Exec.vi"("expected output size  (4096)"=u32 4096, "wait until completion? (T)"=TRUE, "error in (no error)"=w69, "working directory"=w65, "command line"="taskkill /f /im FieldTest.exe") -> ("error out"=w68:errorcluster)  [unwired: 3 in, 3 out]
            }
          }
        }
        frame #4 {
          # "> test.inf"
          # "cmd /c FieldTest.exe testConfig_RfsmOnly.scn"
          n39 = local read "OpenNewFt(T)"() -> (w73:bool)
          n40 = case shown="True" w73 {
            tunnel: w76 -> [w114 w135]
            tunnel: [w114 w134] -> w75
            tunnel: [FALSE TRUE] -> w74
            frame False {
            }
            frame True {
              w115 = " 2>&1"  # string
              n41 = local read "FileName(.txt)"() -> (w123:string)
              n42 = Search/Split String(string=w123, search string/char (-)="." ("regular expression")) -> (substring before match=w124:string)  [unwired: 1 in, 2 out]
              n43 = local read "UseCmdFile(T)"() -> (w128:bool)
              n44 = Concatenate Strings(w124, ".txt" ("string")) -> (w127:string)
              n45 = local read "CmdWindowHide(T)"() -> (w129:bool)
              n46 = local read "working directory"() -> (w122:path)
              n47 = Concatenate Strings("cmd /c FieldTest.exe testConfig_RfsmOnly.scn > " ("command line"), w127, w115) -> (w121:string)
              n48 = Select(t=w121, s=w128, f="cmd /c FieldTest.exe testConfig_RfsmOnly.scn" ("command line")) -> (s? t:f=w118:string)
              "connectToFt" <- w118
              n49 = Build Path(base path=w122, name or relative path=w118) -> (appended path=w120:path)
              n50 = call <vilib>:"System Exec.vi"("expected output size  (4096)"=u32 4096, "run minimized? (F)"=w129, "wait until completion? (T)"=FALSE, "error in (no error)"=w135, "working directory"=w122, "command line"=w118) -> ("error out"=w134:errorcluster, "standard error"=→"cctFt error":string, "standard output"=→"cctFt output":string)  [unwired: 2 in, 1 out]
              n51 = local write "cmd_path_out"(w120) -> ()
            }
          }
          n52 = for {
            N: 3 -> [_]
            tunnel: w74 -> [w85]
            tunnel: [w78] -> w72
            tunnel: w75 -> [w86]
            tunnel: [w84] -> w77
            i -> [w83]
            stop <- w78 stop-if-true
            w79 = 0.0  # f
            w80 = 0.1  # t
            n53 = case shown="True" w85 {
              tunnel: [FALSE ("selection") w97] -> w78
              tunnel: w86 -> [w89 w106]
              tunnel: [w89 w105] -> w87
              frame False {
              }
              frame True {
                w90 = TRUE  # wait until completion? (T)
                w101 = "FieldTest.exe" ("string")
                (unwired) path "C:/" ("working directory")
                # "Check before exiting to make sure FT is open"
                # "FieldTest.exe"
                n54 = local read "working directory"() -> (w91:path)
                n55 = local read "standard output"() -> (w103:string)
                n56 = call <vilib>:"System Exec.vi"("run minimized? (F)"=TRUE, "wait until completion? (T)"=w90, "error in (no error)"=w106, "working directory"=w91, "command line"="tasklist /SVC /FO TABLE") -> ("error out"=w105:errorcluster, "standard output"=w112:string)  [unwired: 3 in, 2 out]
                n57 = call <vilib>:"Trim Whitespace.vi"("string"=w112) -> ("trimmed string"=w102:string)  [unwired: 1 in]
                n58 = Concatenate Strings(w103, w102) -> (w104:string)
                n59 = Match Pattern(string=w102, regular expression=w101) -> (match substring=w107:string, after substring=w95:string)  [unwired: 1 in, 2 out]
                n60 = Search and Replace String(replace all?=TRUE ("replace all? (F)"), input string=w102, search string=w101) -> (number of replacements=w99:i32)  [unwired: 5 in, 3 out]
                n61 = local write "standard output"(w104) -> ()
                n62 = call <vilib>:"Trim Whitespace.vi"("string"=w95) -> ("trimmed string"=w93:string)  [unwired: 1 in]
                n63 = Equal?(x=1, y=w99) -> (x = y?=w96:bool)
                n64 = call <vilib>:"Space Constant.vi"() -> ("String"=w94:string)
                n65 = Match True/False String(2:"INFO: No tasks are running which match the specified criteria." ("false string"), 3:w101, 4:w107) -> (0:w109:bool)  [unwired: 1 out]
                n66 = Search/Split String(string=w93, search string/char (-)=w94) -> (substring before match=w92:string)  [unwired: 1 in, 2 out]
                n67 = And(x=w109, y=w96) -> (x .and. y?=w97:bool)
                n68 = local write "PID"(w92) -> ()
              }
            }
            n69 = Greater Than 0?(x=w83) -> (x > 0?=w81:bool)
            n70 = Select(t=w80, s=w81, f=w79) -> (s? t:f=w82:dbl)
            n71 = call <vilib>:"High Resolution Polling Wait.vi"("error in (no error)"=w87, "seconds to wait"=w82) -> ("error out"=w84:errorcluster)  [unwired: 9 in]
          }
          "success?(t)" <- w72
        }
      }
    }
    frame True {
    }
  }
  "error out" <- w3
